vi "add and multip.vi"(8 "error in (no error)":errorcluster, 10 "y":dbl, 11 "x":dbl) -> (0 "error out":errorcluster, 2 "result":dbl)   [LabVIEW 2011]
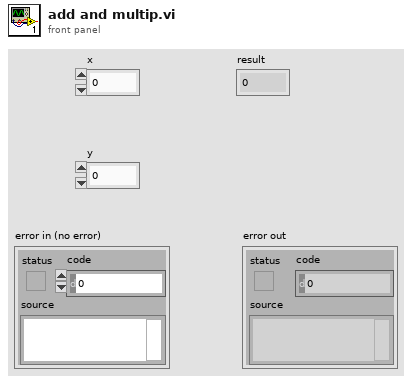
[diagram p1: front panel]
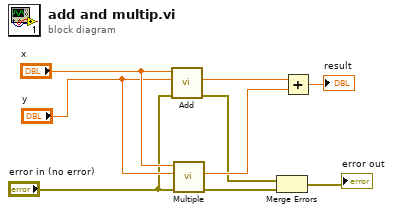
[diagram p0: block diagram]
diagram:
  n1 = call "Add.vi"("error in (no error)"="error in (no error)", "input2"="y", "input1"="x") -> ("error out"=w2:errorcluster, "output"=w8:dbl)  [unwired: 7 in]
  n2 = call "Multiple.vi"("error in (no error)"="error in (no error)", "input2"="y", "input1"="x") -> ("error out"=w1:errorcluster, "output"=w7:dbl)  [unwired: 7 in]
  n3 = Merge Errors(w2, w1) -> (→"error out":errorcluster)
  n4 = Add(x=w8, y=w7) -> (x+y=→"result":dbl)
